vi "picoquant_plot_histogram.vi"(8 "error in (no error)":errorcluster, 9 "initialize_histogram?":bool, 10 "data":T1, 11 "picoquant_generic in":refnum<class "picoquant_generic.lvclass">) -> (0 "error out":errorcluster, 2 "histogram":cluster{"Axis":dbl[], "Histogram":i32[]}, 3 "picoquant_generic out":refnum<class "picoquant_generic.lvclass">)   [LabVIEW 2015, in "picoquant_generic.lvclass"]
uses:
  picoquant_generic.lvclass
  picoquant_data_tdef.ctl
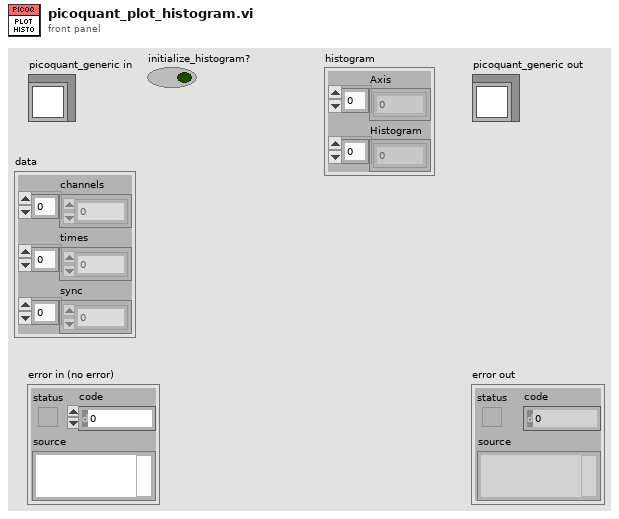
[diagram p1: front panel]
types:
  T1 = typedef "picoquant_data_tdef.ctl" = cluster{"channels":u8[], "times":u64[], "sync":u64[]}
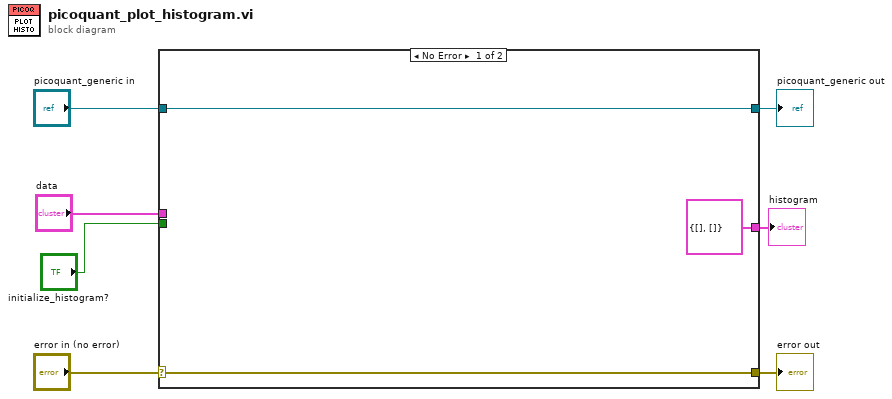
[diagram p0: block diagram]
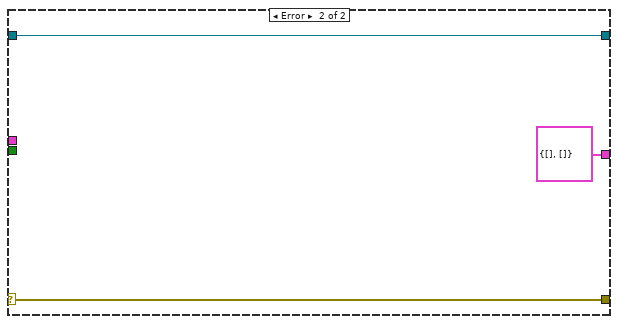
[diagram p2: hidden frame]
diagram:
  n1 = case shown="No Error" "error in (no error)" {
    selector: "error in (no error)" -> [w9 w13]
    tunnel: [w9 w13] -> w6
    tunnel: [w10 w12] -> w4
    tunnel: "picoquant_generic in" -> [w10 w12]
    tunnel: "data" -> [_ _]
    tunnel: "initialize_histogram?" -> [_ _]
    tunnel: [cluster{"Axis":dbl[], "Histogram":i32[]} {"Axis"=[], "Histogram"=[]} cluster{"Axis":dbl[], "Histogram":i32[]} {"Axis"=[], "Histogram"=[]}] -> w1
    frame No Error {
    }
    frame Error {
    }
  }
  "error out" <- w6
  "picoquant_generic out" <- w4
  "histogram" <- w1
